vi "create.AddOrderExpanded.vi"(8 "error in":errorcluster, 10 "AddOrderExpanded.Parameters":T1, 11 "AddOrderTest in":refnum<class "AddOrderExpanded.lvclass">) -> (0 "error out":errorcluster, 3 "AddOrderTest out":refnum<class "AddOrderExpanded.lvclass">)   [LabVIEW 2020, in "AddOrderExpanded.lvclass"]
uses:
  AddOrderExpanded.lvclass
  AddOrderExpanded.Parameters.ctl
  FieldSpec.ctl
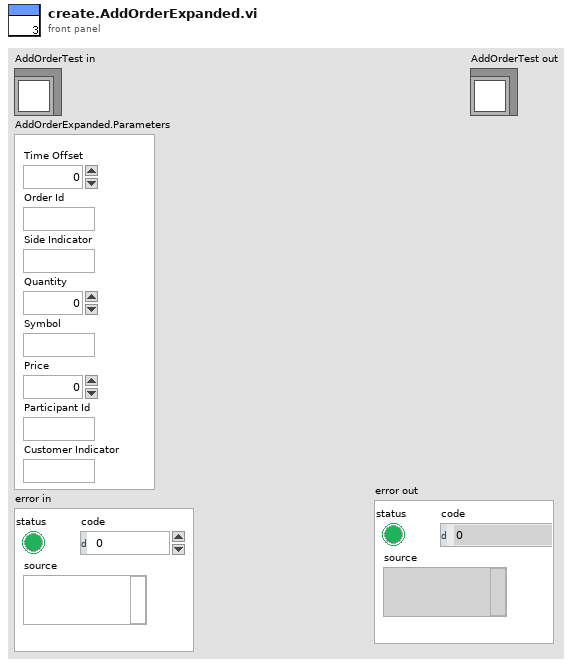
[diagram p1: front panel]
types:
  T1 = typedef "AddOrderExpanded.lvclass/AddOrderExpanded.Parameters.ctl" = cluster{"Time Offset":u32, "Order Id":string, "Quantity":u32, "Symbol":string, "Side Indicator":string, "Price":dbl, "Participant Id":string, "Customer Indicator":string}
  T2 = typedef "FieldSpec.ctl" = cluster{"Name":string, "Offset":i32, "Length":i32, "FieldType":enum16{"Alphanumeric", "Binary", "BinaryLongPrice", "BinaryShortPrice", "BitField", "PrintableAscii", "Value"}, "FieldValue":variant}
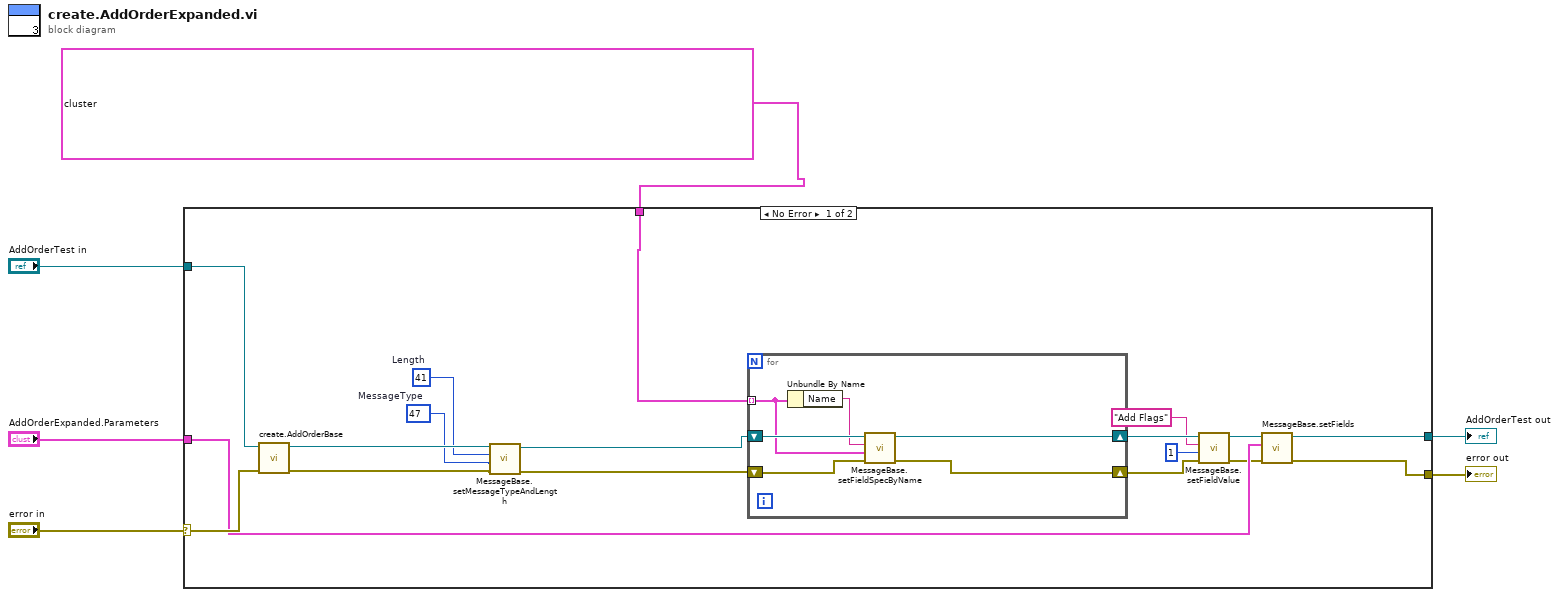
[diagram p0: block diagram]
diagram:
  n1 = case shown="No Error" "error in" {
    selector: "error in" -> [w17 w32]
    tunnel: [w14 w32] -> w5
    tunnel: [w13 w31] -> w3
    tunnel: "AddOrderTest in" -> [w18 w31]
    tunnel: "AddOrderExpanded.Parameters" -> [w16 _]
    tunnel: T2[] [{"Name"="Symbol", "Offset"=19, "Length"=8, "FieldType"=enum."PrintableAscii", "FieldValue"=variant}, {"Name"="Price", "Offset"=27, "Length"=8, "FieldType"=enum."BinaryLongPrice", "FieldValue"=variant}, {"Name"="Add Flags", "Offset"=35, "Length"=1, "FieldType"=enum."BitField", "FieldValue"=variant}, {"Name"="Participant Id", "Offset"=36, "Length"=4, "FieldType"=enum."Alphanumeric", "FieldValue"=variant}, {"Name"="Customer Indicator", "Offset"=40, "Length"=1, "FieldType"=enum."Alphanumeric", "FieldValue"=variant}] ("appended array") -> [w15 _]
    frame No Error {
      w23 = u8 47  # MessageType
      w22 = u8 41  # Length
      n2 = call-dynamic "create.AddOrderBase.vi"("error in (no error)"=w17, "AddOrderBase in"=w18) -> ("error out"=w21:errorcluster, "AddOrderBase out"=w24:refnum<class "AddOrderExpanded.lvclass">)  [unwired: 8 in]
      n3 = call-dynamic "MessageBase.setMessageTypeAndLength.vi"("error in (no error)"=w21, "MessageType"=w23, "Length"=w22, "MessageBase in"=w24) -> ("error out"=w20:errorcluster, "MessageBase out"=w19:refnum<class "AddOrderExpanded.lvclass">)  [unwired: 6 in]
      n4 = for {
        tunnel: w15 -> [w27] mode=indexing
        shift-right: [w26] -> w10
        shift-left: w19 -> [w30]
        shift-right: [w25] -> w7
        shift-left: w20 -> [w29]
        n5 = Unbundle By Name(w27) -> ("Name"=w28:string)
        n6 = call-dynamic "MessageBase.setFieldSpecByName.vi"("error in (no error)"=w29, "FIeldSpec"=w27, "Field.Name"=w28, "MessageBase in"=w30) -> ("error out"=w25:errorcluster, "MessageBase out"=w26:refnum<class "AddOrderExpanded.lvclass">)  [unwired: 6 in]
      }
      n7 = call-dynamic "MessageBase.setFieldValue.vi"("error in (no error)"=w7, "Value"=u8 1, "FIeld.Name"="Add Flags", "MessageBase in"=w10) -> ("error out"=w12:errorcluster, "MessageBase out"=w11:refnum<class "AddOrderExpanded.lvclass">)  [unwired: 6 in]
      n8 = call-dynamic "MessageBase.setFields.vi"("error in (no error)"=w12, "Cluster (dup)"=w16, "MessageBase in"=w11) -> ("error out"=w14:errorcluster, "MessageBase out"=w13:refnum<class "AddOrderExpanded.lvclass">)  [unwired: 7 in]
    }
    frame Error {
    }
  }
  "error out" <- w5
  "AddOrderTest out" <- w3
